vi "CCD photon image_Shaowei.vi"() -> ()   [LabVIEW 2009]
uses:
  <vilib>/Utility/file.llb/Read From Spreadsheet File (DBL).vi
  Instance           5 35Saved   CCD photon image_540_800_CR .vi
  Instance           4 35Saved   CCD photon image_540_800_CR .vi
  Instance           3 35Saved   CCD photon image_540_800_CR .vi
  Instance           8 35Saved   CCD photon image_540_800_CR .vi
  <vilib>/Analysis/Matrix/Numeric/Conversions/Array To Matrix - RA2.vi
  Instance          12 35Saved   CCD photon image_540_800_CR .vi
  Instance          18 35Saved   CCD photon image_540_800_CR .vi
  <vilib>/Analysis/Matrix/NI_Matrix.lvlib
panel:
  in  "Save Matrix6":bool
  in  "Save Matrix5":bool
  in  "Save Matrix3":bool
  in  "Save Matrix4":bool
  out "Matrix 2":string
  in  "Save Matrix2":bool
  out "Matrix 1":string
  in  "Save Matrix1":bool
  in  "select 2":bool
  in  "select":bool
  in  "next 2":bool
  in  "next":bool
  in  "previous 2":bool
  in  "previous":bool
  in  "?":bool
  out "?":path
  out "?":path
  out "?":i32
  in  "?":bool
  in  "stop 2":bool
  in  "#6":bool
  in  "#5":bool
  in  "to":dbl=950.0
  in  "From":dbl=550.0
  out "Intensity Graph 6":dbl[][](graph)
  out "Col":dbl
  out "to":dbl
  out "Matrix 6":string
  in  "lstart (nm)":dbl
  in  "lend (nm)":dbl
  out "eV":dbl
  out "eV":dbl
  out "Intensity Graph 5":dbl[][](graph)
  out "Col":dbl
  out "to":dbl
  out "Matrix 5":string
  in  "lstart (nm)":dbl
  in  "lend (nm)":dbl
  out "eV":dbl
  out "eV":dbl
  in  "?":bool
  out "MAX":dbl
  out "MIN":dbl
  out "X":sgl
  out "Y":sgl
  out "to":dbl
  out "Col":dbl
  out "eV":dbl
  out "eV":dbl
  in  "lend (nm)":dbl
  in  "lstart (nm)":dbl
  out "eV":dbl
  out "eV":dbl
  in  "lend (nm)":dbl
  in  "lstart (nm)":dbl
  out "to":dbl
  out "Col":dbl
  out "to":dbl
  out "Col":dbl
  out "eV":dbl
  out "eV":dbl
  in  "lend (nm)":dbl
  in  "lstart (nm)":dbl
  in  "?":dbl=32.0
  out "eV":dbl
  out "eV":dbl
  in  "lend (nm)":dbl
  in  "lstart (nm)":dbl
  out "to":dbl
  out "Col":dbl
  in  "#3":bool
  in  "#4":bool
  in  "#2":bool
  out "Intensity Graph 4":dbl[][](graph)
  out "Matrix 4":string
  out "Intensity Graph 3":dbl[][](graph)
  out "Matrix 3":string
  out "Intensity Graph 2":dbl[][](graph)
  out "Intensity Graph":dbl[][](graph)
  # "Input File"
  # "2 Files"
  # "1 File"
  # "1st"
  # "2nd"
  # "Spectra Range"
  # "nm"
  # "nm"
  # "# of Pixel"
  # "Image Size"
  # "Bit"
  # "Active Matrix"
  # "ON"
  # "OFF"
  # "Cosmic Ray Removal"
  # "NO"
  # "YES"
  # "Value"
  # "Position"
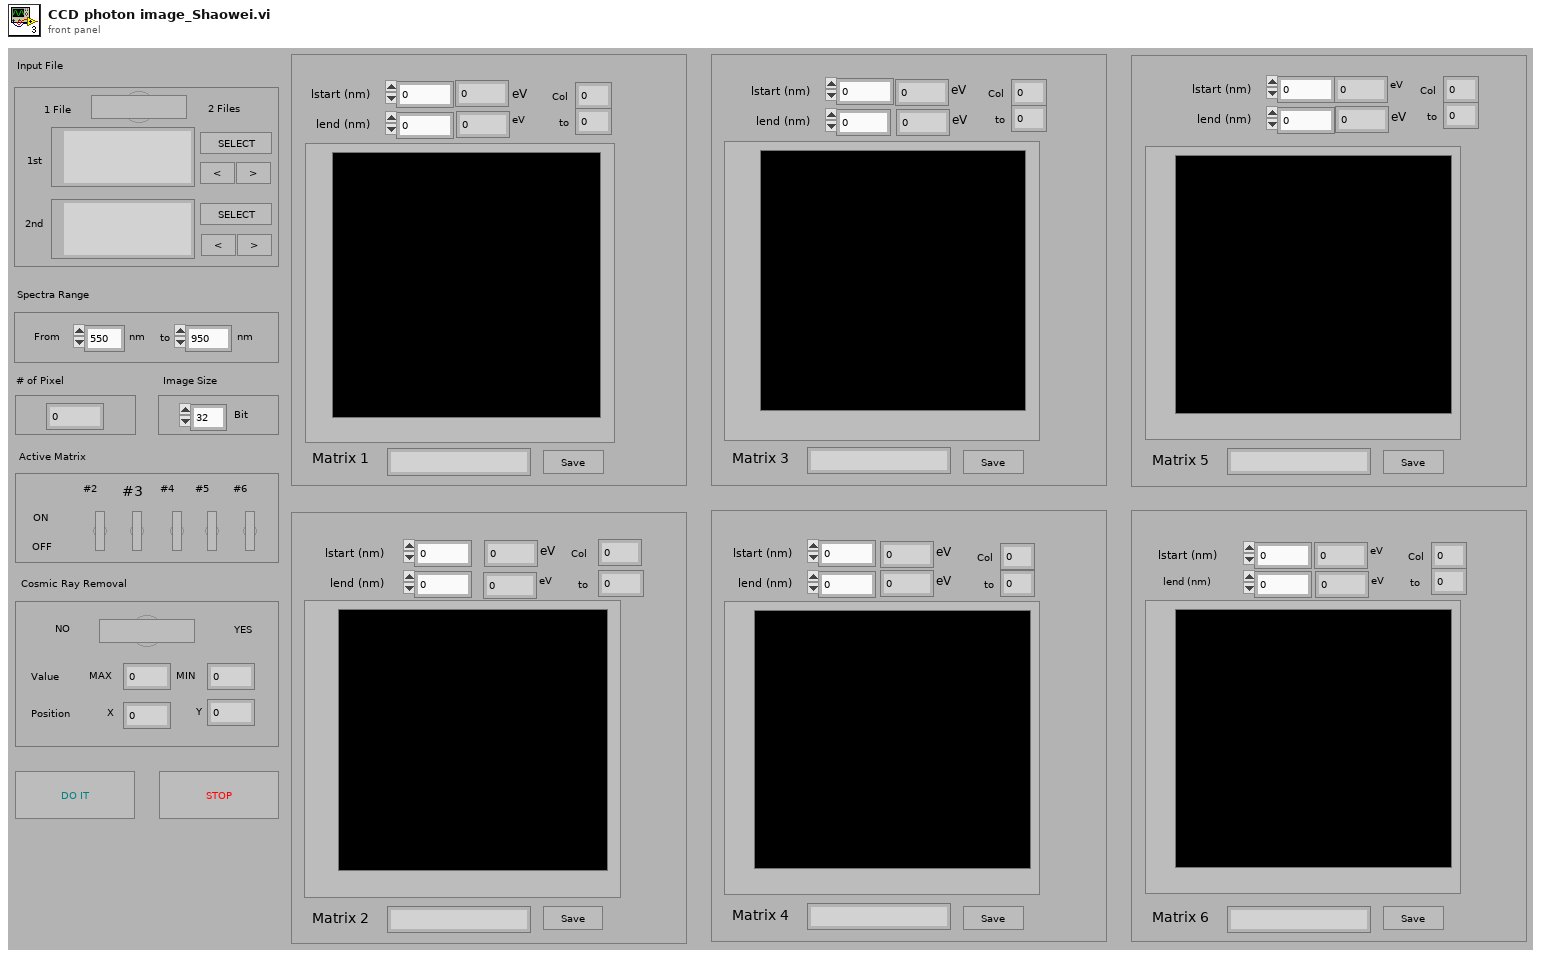
[diagram p1: front panel]
types:
  T1 = typedef "NI_Matrix.lvlib/RealMatrix.ctl" = dbl[][]
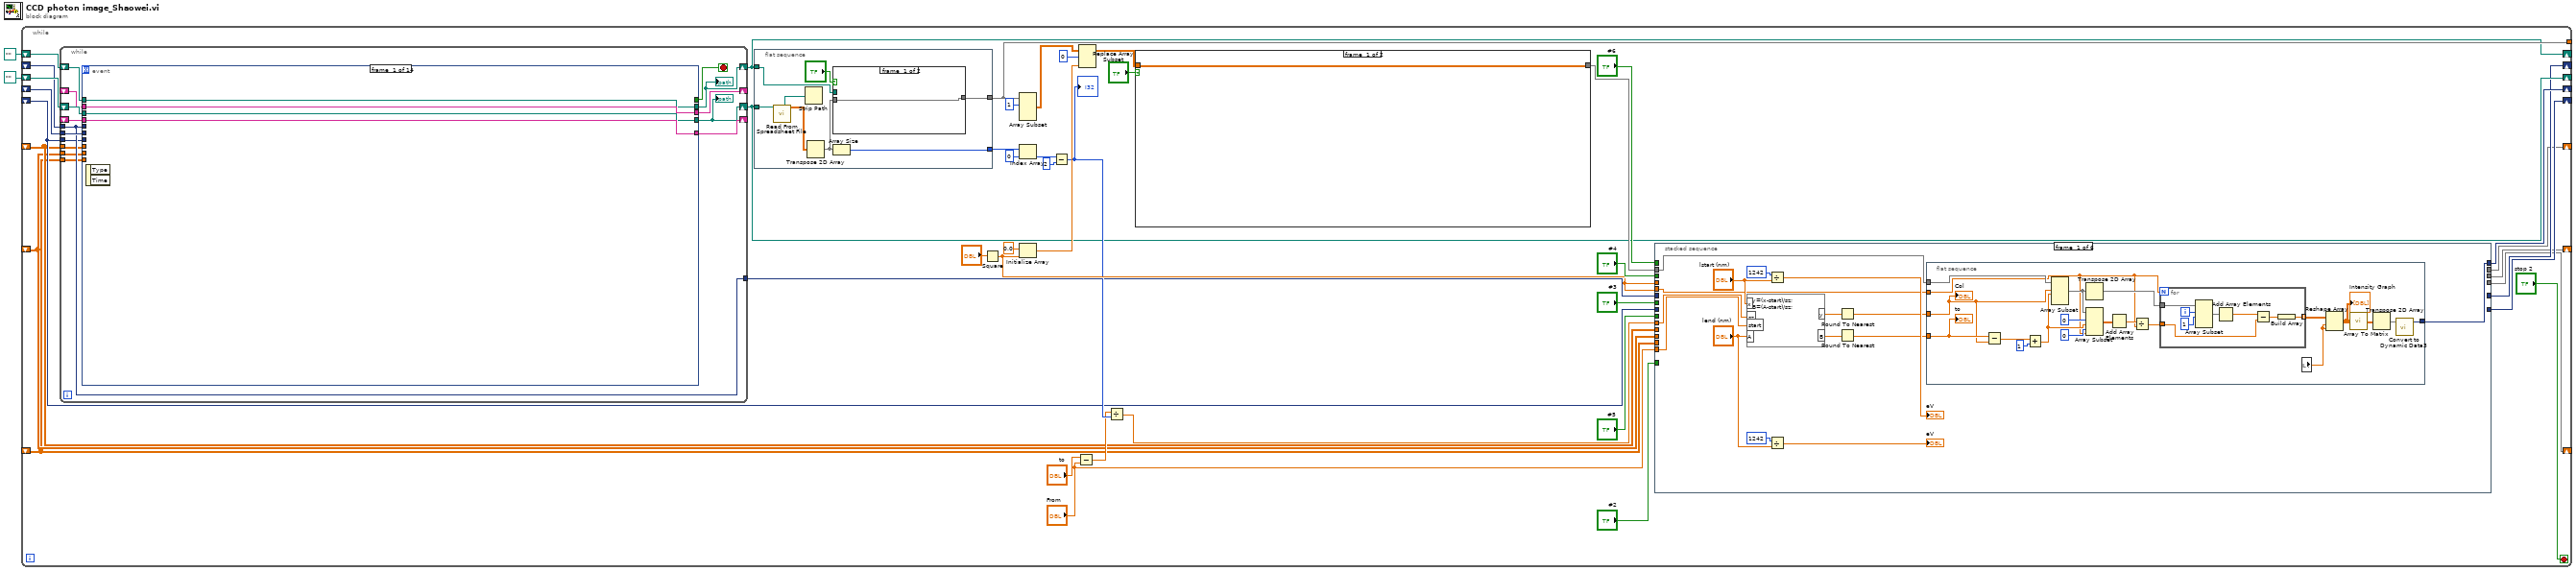
[diagram p0: block diagram]
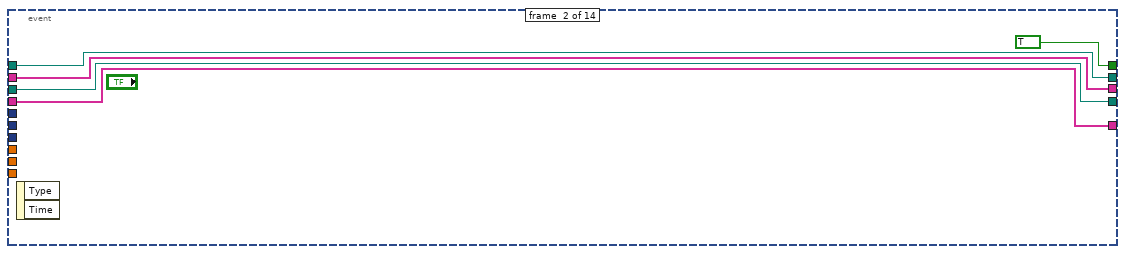
[diagram p2: hidden frame]
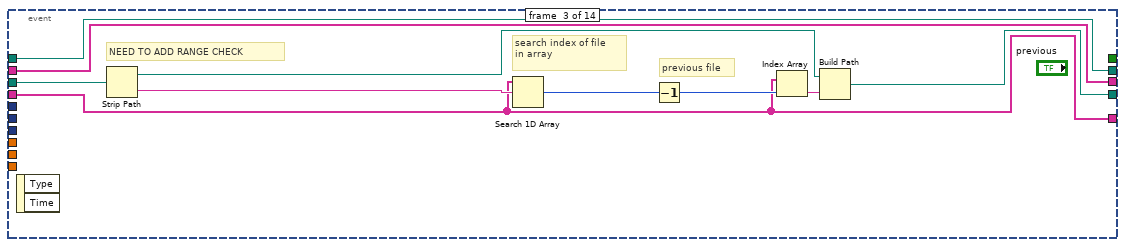
[diagram p3: hidden frame]
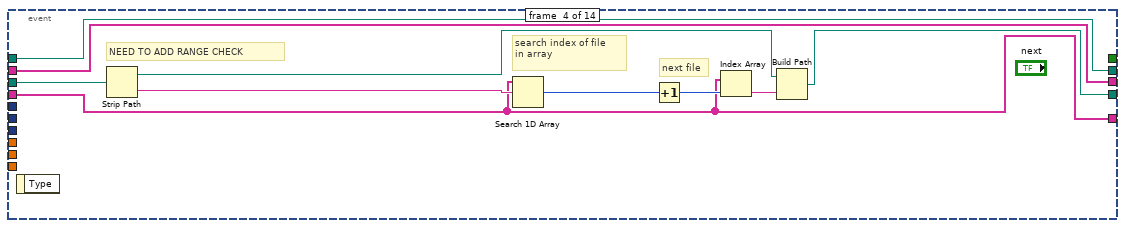
[diagram p4: hidden frame]
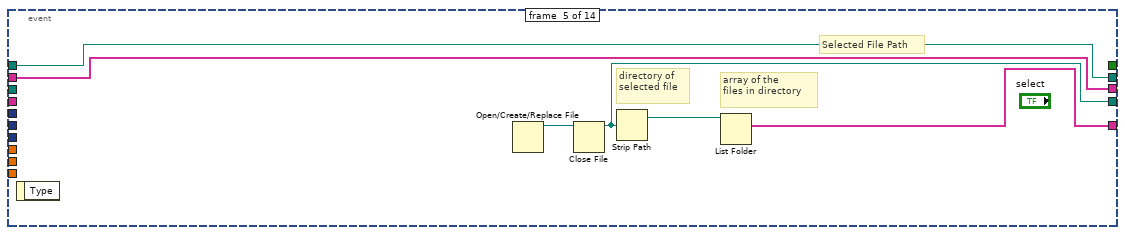
[diagram p5: hidden frame]
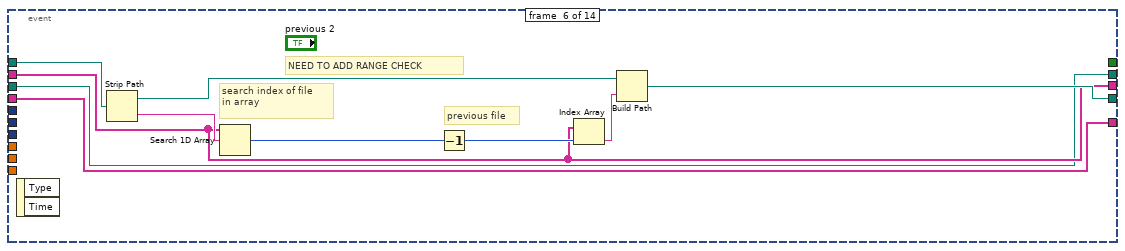
[diagram p6: hidden frame]
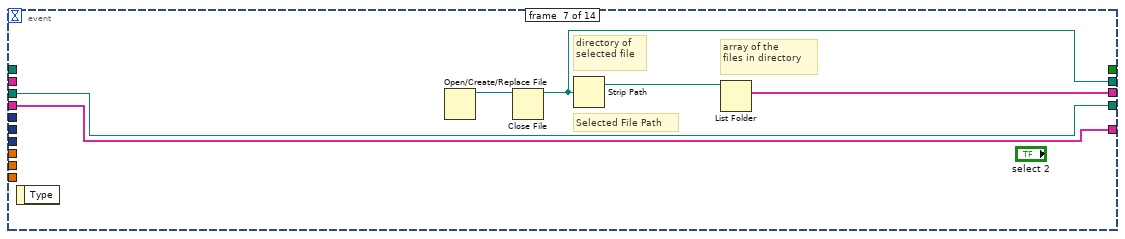
[diagram p7: hidden frame]
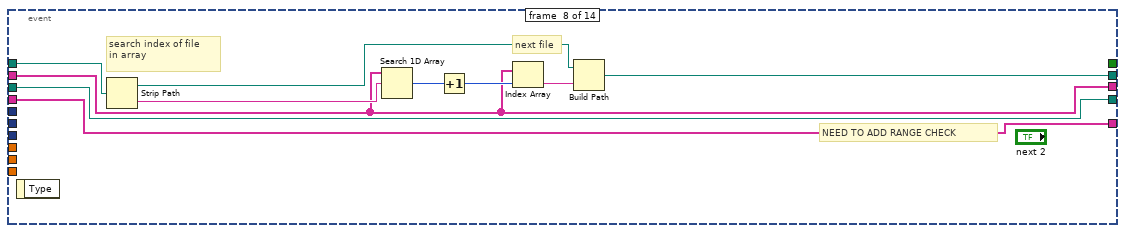
[diagram p8: hidden frame]
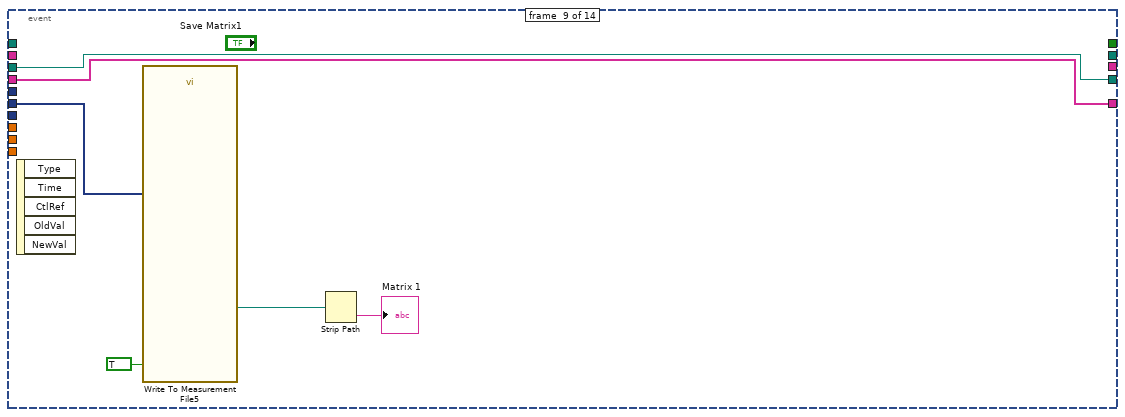
[diagram p9: hidden frame]
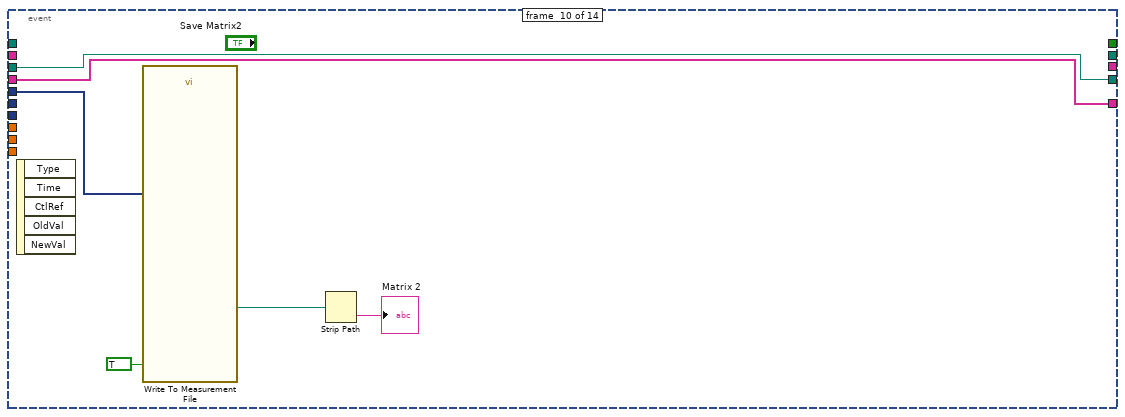
[diagram p10: hidden frame]
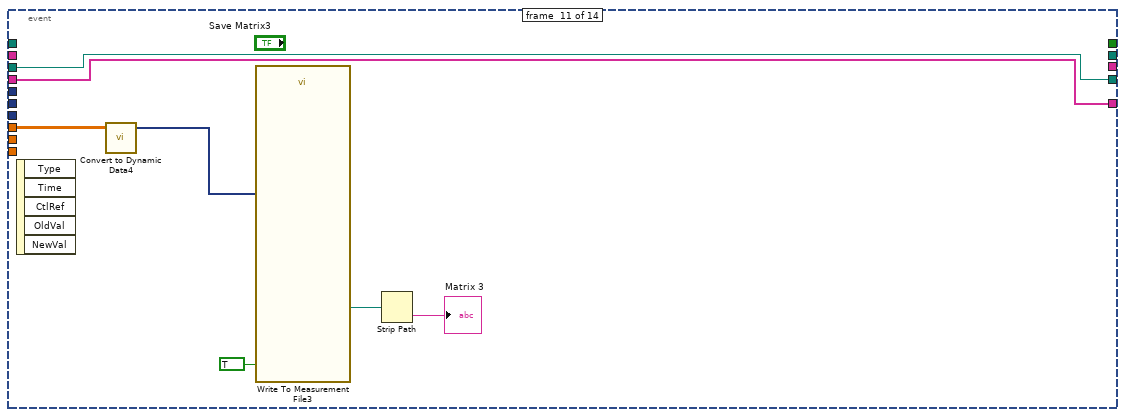
[diagram p11: hidden frame]
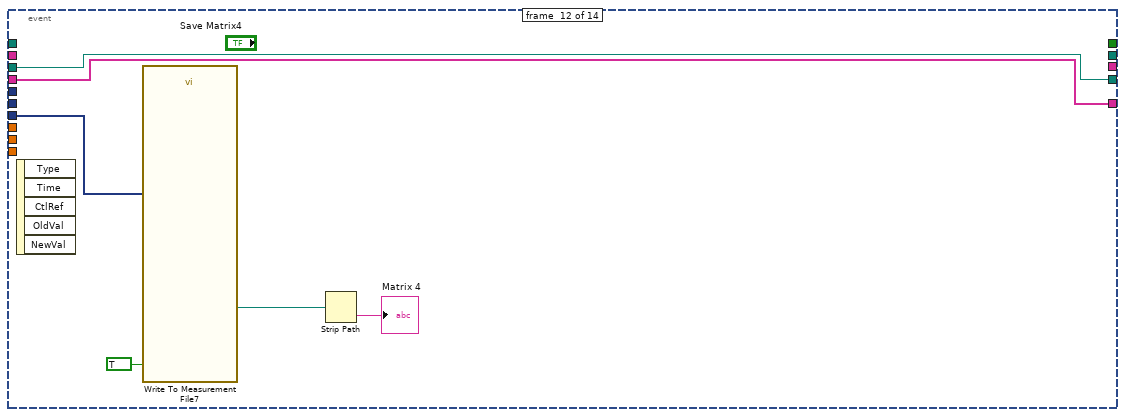
[diagram p12: hidden frame]
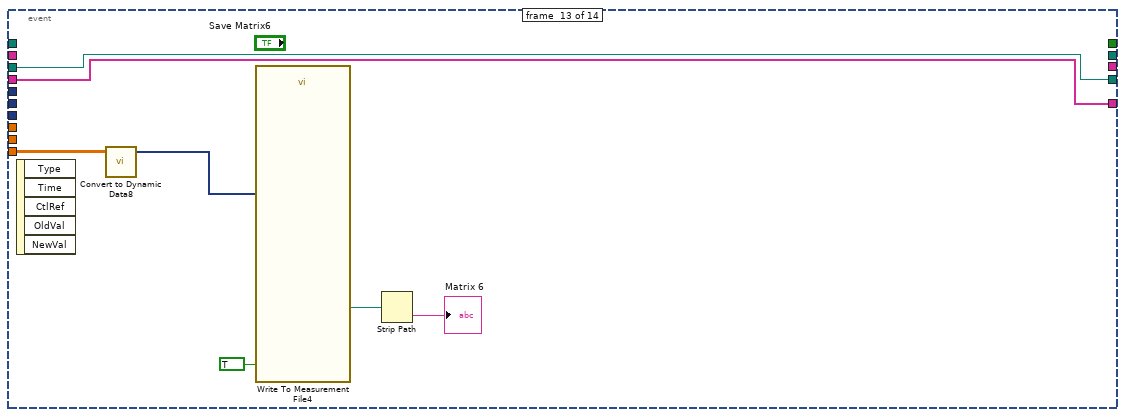
[diagram p13: hidden frame]
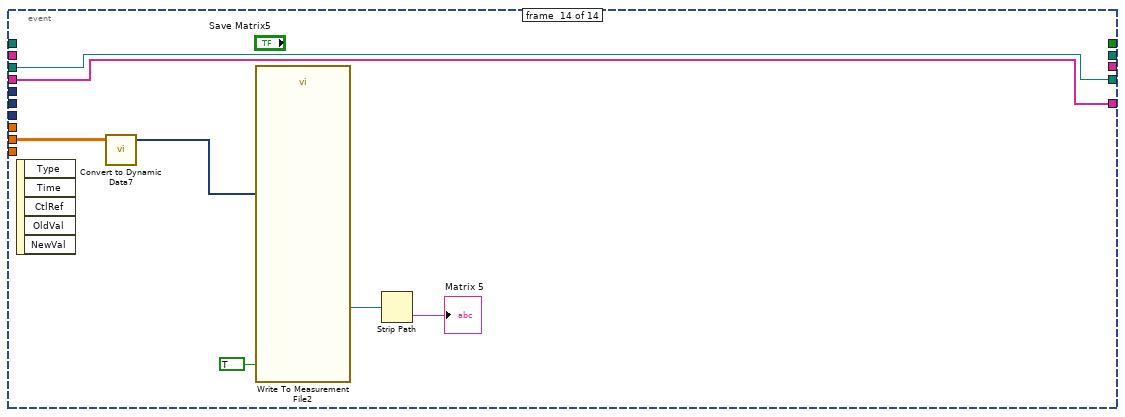
[diagram p14: hidden frame]
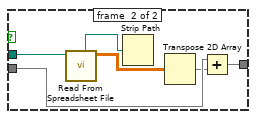
[diagram p15: hidden frame]
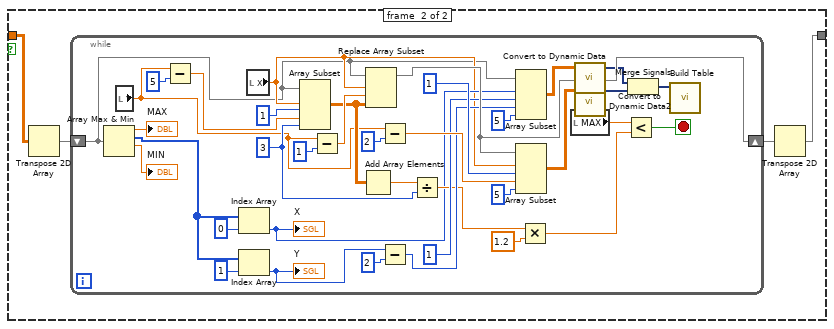
[diagram p16: hidden frame]
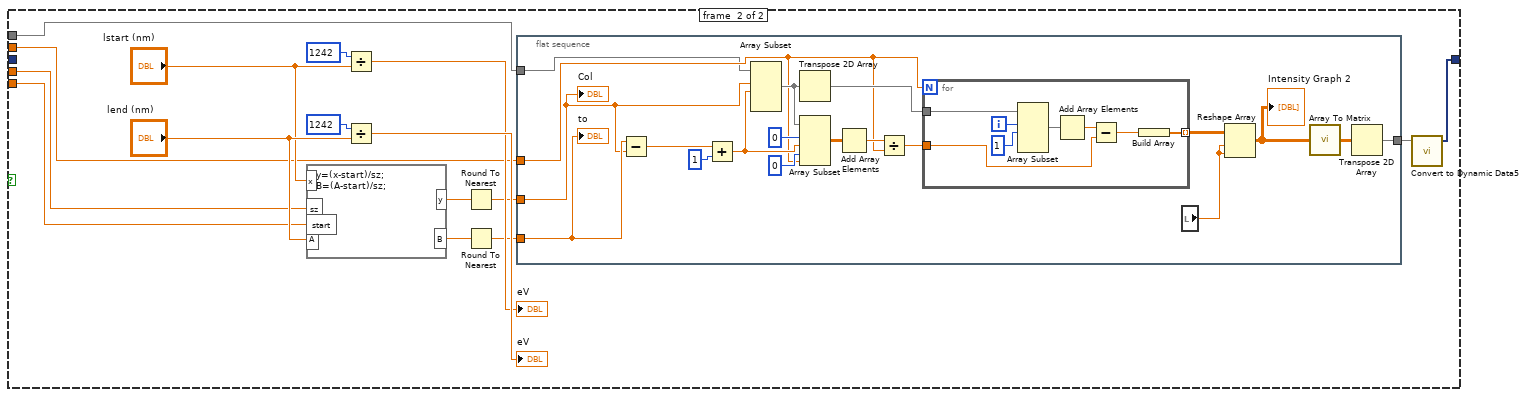
[diagram p18: hidden frame]
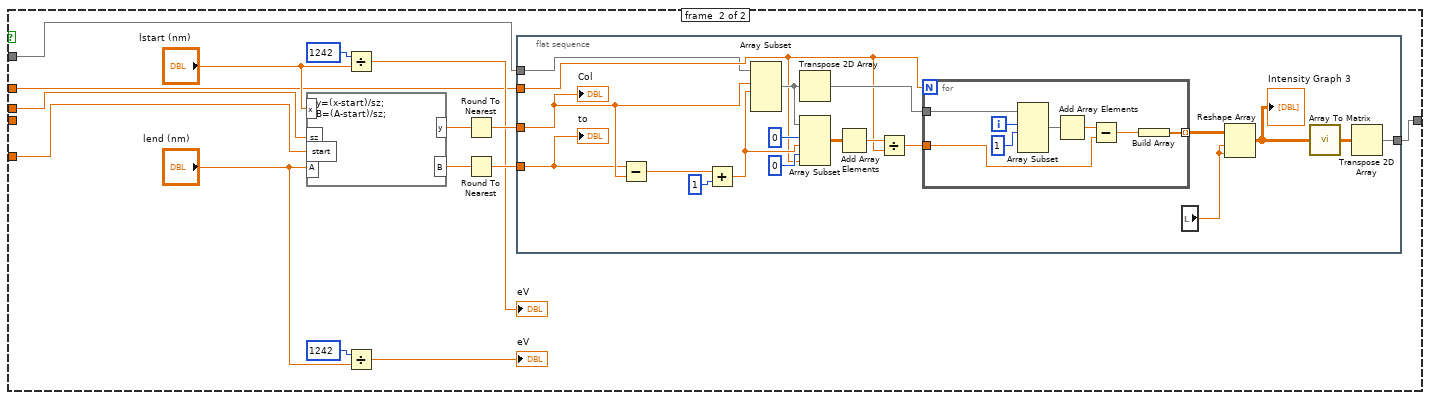
[diagram p20: hidden frame]
diagram:
  n1 = while {
    tunnel: [w26] -> _
    shift-right: [w16] -> _
    shift-left: path "" ("path") -> [w18]
    shift-right: [w17] -> _
    shift-left: path "" ("path") -> [w19]
    shift-right: [w15] -> _
    shift-left: _ -> [w14]
    shift-right: [w13] -> _
    shift-left: _ -> [w12]
    shift-right: [w10] -> _
    shift-left: _ -> [w9]
    shift-right: [w8] -> _
    shift-left: _ -> [w7]
    shift-right: [w6] -> _
    shift-left: _ -> [w5]
    shift-right: [w4] -> _
    shift-left: _ -> [w3]
    stop <- "stop 2" stop-if-true
    n2 = while {
      shift-right: [w60] -> _
      shift-left: _ -> [w59]
      shift-right: [w52] -> w16
      shift-left: w18 -> [w58]
      shift-right: [w57] -> w17
      shift-left: w19 -> [w56]
      shift-right: [w55] -> _
      shift-left: _ -> [w54]
      tunnel: w14 -> [w51]
      tunnel: w12 -> [w50]
      tunnel: [w50] -> w11
      tunnel: w9 -> [w49]
      tunnel: w7 -> [w48]
      tunnel: w5 -> [w47]
      tunnel: w3 -> [w46]
      stop <- w53 stop-if-true
      n3 = event shown="[12] \"Save Matrix6\": Value Change" {
        selector: _ -> [_ _ _ _ _ _ _ _ _ _ _ _ _ _]
        dyn-events: _ -> [_ _ _ _ _ _ _ _ _ _ _ _ _ _]
        timeout: _ -> [_ _ _ _ _ _ _ _ _ _ _ _ _ _]
        tunnel: [_ TRUE _ _ _ _ _ _ _ _ _ _ _ _] -> w53
        tunnel: [w63 w67 w72 w84 w92 w100 w107 w113 w127 w133 w140 w146 w153 w160] -> w52
        tunnel: [w64 w68 w74 w82 w93 w97 w106 w112 w126 w132 w139 w145 w152 w159] -> w60
        tunnel: w59 -> [w64 w68 w74 w82 _ w97 w106 w112 w126 w132 w139 w145 w152 w159]
        tunnel: w58 -> [w63 w67 w79 w83 _ w96 w107 w113 w127 w133 w140 w146 w153 w160]
        tunnel: [w61 w65 w70 w80 w90 w96 w109 w114 _ _ _ _ _ _] -> w57
        tunnel: w56 -> [w61 w65 w70 w80 w90 w99 _ w115 _ _ _ _ _ _]
        tunnel: [w62 w66 w71 w81 w91 w98 w108 w116 _ _ _ _ _ _] -> w55
        tunnel: w54 -> [w62 w66 w71 w81 w91 w98 _ w116 _ _ _ _ _ _]
        tunnel: w51 -> [_ _ _ _ _ _ _ _ w125 _ _ _ _ _]
        tunnel: w50 -> [_ _ _ _ _ _ _ _ _ w131 _ _ _ _]
        tunnel: w49 -> [_ _ _ _ _ _ _ _ _ _ _ w141 _ _]
        tunnel: w48 -> [_ _ _ _ _ _ _ _ _ _ w135 _ _ _]
        tunnel: w47 -> [_ _ _ _ _ _ _ _ _ _ _ _ _ w156]
        tunnel: w46 -> [_ _ _ _ _ _ _ _ _ _ _ _ w148 _]
        event #0 {
          n4 = event-data() -> ()  [unwired: 1 in, 2 out]
        }
        event #1 {
          n5 = event-data() -> ()  [unwired: 1 in, 2 out]
        }
        event #2 {
          # "NEED TO ADD RANGE CHECK"
          # "previous file"
          # "search index of file\nin array"
          n6 = event-data() -> ()  [unwired: 1 in, 2 out]
          n7 = Strip Path(path=w79) -> (stripped path=w76:path, name=w78:string)
          n8 = Search 1D Array(1D array=w74, element=w78) -> (index of element=w77:i32)  [unwired: 1 in]
          n9 = Decrement(x=w77) -> (x-1=w75:i32)
          n10 = Index Array(array=w74, index=w75) -> (element=w73:string)
          n11 = Build Path(base path=w76, name or relative path=w73) -> (appended path=w72:path)
        }
        event #3 {
          # "NEED TO ADD RANGE CHECK"
          # "next file"
          # "search index of file\nin array"
          n12 = event-data() -> ()  [unwired: 1 in, 1 out]
          n13 = Strip Path(path=w83) -> (stripped path=w87:path, name=w89:string)
          n14 = Search 1D Array(1D array=w82, element=w89) -> (index of element=w88:i32)  [unwired: 1 in]
          n15 = Increment(x=w88) -> (x+1=w86:i32)
          n16 = Index Array(array=w82, index=w86) -> (element=w85:string)
          n17 = Build Path(base path=w87, name or relative path=w85) -> (appended path=w84:path)
        }
        event #4 {
          # "array of the \nfiles in directory"
          # "directory of\nselected file"
          # "Selected File Path"
          n18 = event-data() -> ()  [unwired: 1 in, 1 out]
          n19 = Open/Create/Replace File() -> (refnum out=w95:refnum<file>)  [unwired: 6 in, 2 out]
          n20 = Close File(refnum=w95) -> (path=w92:path)  [unwired: 1 in, 1 out]
          n21 = Strip Path(path=w92) -> (stripped path=w94:path)  [unwired: 1 out]
          n22 = List Folder(path=w94) -> (filenames=w93:string[])  [unwired: 3 in, 3 out]
        }
        event #5 {
          # "NEED TO ADD RANGE CHECK"
          # "previous file"
          # "search index of file\nin array"
          n23 = event-data() -> ()  [unwired: 1 in, 2 out]
          n24 = Strip Path(path=w99) -> (stripped path=w103:path, name=w105:string)
          n25 = Search 1D Array(1D array=w98, element=w105) -> (index of element=w104:i32)  [unwired: 1 in]
          n26 = Decrement(x=w104) -> (x-1=w102:i32)
          n27 = Index Array(array=w98, index=w102) -> (element=w101:string)
          n28 = Build Path(base path=w103, name or relative path=w101) -> (appended path=w100:path)
        }
        event #6 {
          # "array of the \nfiles in directory"
          # "directory of\nselected file"
          # "Selected File Path"
          n29 = event-data() -> ()  [unwired: 1 in, 1 out]
          n30 = Open/Create/Replace File() -> (refnum out=w111:refnum<file>)  [unwired: 6 in, 2 out]
          n31 = Close File(refnum=w111) -> (path=w109:path)  [unwired: 1 in, 1 out]
          n32 = Strip Path(path=w109) -> (stripped path=w110:path)  [unwired: 1 out]
          n33 = List Folder(path=w110) -> (filenames=w108:string[])  [unwired: 3 in, 3 out]
        }
        event #7 {
          # "NEED TO ADD RANGE CHECK"
          # "next file"
          # "search index of file\nin array"
          n34 = event-data() -> ()  [unwired: 1 in, 1 out]
          n35 = Strip Path(path=w115) -> (stripped path=w119:path, name=w121:string)
          n36 = Search 1D Array(1D array=w116, element=w121) -> (index of element=w120:i32)  [unwired: 1 in]
          n37 = Increment(x=w120) -> (x+1=w118:i32)
          n38 = Index Array(array=w116, index=w118) -> (element=w117:string)
          n39 = Build Path(base path=w119, name or relative path=w117) -> (appended path=w114:path)
        }
        event #8 {
          n40 = event-data() -> ()  [unwired: 1 in, 5 out]
          n41 = call "Write To Measurement File5"("Signals"=w125, "Reset"=TRUE) -> ("Filename Out"=w123:path)  [unwired: 15 in, 2 out]
          n42 = Strip Path(path=w123) -> (name=→"Matrix 1":string)  [unwired: 1 out]
        }
        event #9 {
          n43 = event-data() -> ()  [unwired: 1 in, 5 out]
          n44 = call "Write To Measurement File"("Signals"=w131, "Reset"=TRUE) -> ("Filename Out"=w129:path)  [unwired: 15 in, 2 out]
          n45 = Strip Path(path=w129) -> (name=→"Matrix 2":string)  [unwired: 1 out]
        }
        event #10 {
          n46 = event-data() -> ()  [unwired: 1 in, 5 out]
          n47 = call "Convert to Dynamic Data4"("2D Array"=w135) -> ("Dynamic Data Type"=w134:dynamicdata)  [unwired: 3 in]
          n48 = call "Write To Measurement File3"("Signals"=w134, "Reset"=TRUE) -> ("Filename Out"=w138:path)  [unwired: 15 in, 2 out]
          n49 = Strip Path(path=w138) -> (name=→"Matrix 3":string)  [unwired: 1 out]
        }
        event #11 {
          n50 = event-data() -> ()  [unwired: 1 in, 5 out]
          n51 = call "Write To Measurement File7"("Signals"=w141, "Reset"=TRUE) -> ("Filename Out"=w143:path)  [unwired: 15 in, 2 out]
          n52 = Strip Path(path=w143) -> (name=→"Matrix 4":string)  [unwired: 1 out]
        }
        event #12 {
          n53 = event-data() -> ()  [unwired: 1 in, 5 out]
          n54 = call "Convert to Dynamic Data8"("2D Array"=w148) -> ("Dynamic Data Type"=w147:dynamicdata)  [unwired: 3 in]
          n55 = call "Write To Measurement File4"("Signals"=w147, "Reset"=TRUE) -> ("Filename Out"=w150:path)  [unwired: 15 in, 2 out]
          n56 = Strip Path(path=w150) -> (name=→"Matrix 6":string)  [unwired: 1 out]
        }
        event #13 {
          n57 = event-data() -> ()  [unwired: 1 in, 5 out]
          n58 = call "Convert to Dynamic Data7"("2D Array"=w156) -> ("Dynamic Data Type"=w155:dynamicdata)  [unwired: 3 in]
          n59 = call "Write To Measurement File2"("Signals"=w155, "Reset"=TRUE) -> ("Filename Out"=w157:path)  [unwired: 15 in, 2 out]
          n60 = Strip Path(path=w157) -> (name=→"Matrix 5":string)  [unwired: 1 out]
        }
      }
      "?" <- w52
      "?" <- w57
    }
    n61 = flat-sequence {
      tunnel: [w167] -> w26
      tunnel: [w164] -> w23
      tunnel: w16 -> [w162]
      tunnel: w17 -> [w161]
      frame #0 {
        n62 = call-poly <vilib>:"Read From Spreadsheet File.vi"("file path (dialog if empty)"=w162) -> ("all rows"=w165:dbl[][], "new file path (Not A Path if cancelled)"=w168:path)  [unwired: 6 in, 3 out]
        n63 = Strip Path(path=w168) -> ()  [unwired: 2 out]
        n64 = Transpose 2D Array(2D array=w165) -> (transposed array=w163:dbl[][])
        n65 = case shown="False" "?" {
          tunnel: w163 -> [w169 w174]
          tunnel: [w169 w173] -> w167
          tunnel: w161 -> [_ w170]
          frame #0 {
          }
          frame #1 {
            n66 = call-poly <vilib>:"Read From Spreadsheet File.vi"("file path (dialog if empty)"=w170) -> ("all rows"=w172:dbl[][], "new file path (Not A Path if cancelled)"=w175:path)  [unwired: 6 in, 3 out]
            n67 = Strip Path(path=w175) -> ()  [unwired: 2 out]
            n68 = Transpose 2D Array(2D array=w172) -> (transposed array=w171:dbl[][])
            n69 = Add(x=w174, y=w171) -> (x+y=w173:dbl[][])
          }
        }
        n70 = Array Size(array=w163) -> (size(s)=w164:i32[])
      }
    }
    n71 = Square(x="?") -> (x^2=w37:dbl)
    n72 = Array Subset(array=w26, index (row)=1) -> (w39:dbl[][])  [unwired: 3 in]
    n73 = Index Array(array=w23, index=0) -> (element=w21:i32)
    n74 = Initialize Array(0.0 ("element"), w37) -> (w41:dbl[])
    n75 = Subtract(x=w21, y=2) -> (x-y=w33:i32)
    "?" <- w33
    n76 = Subtract(x="to", y="From") -> (x-y=w32:dbl)
    n77 = Replace Array Subset(array=w39, new element=w41, index (row)=0) -> (w36:dbl[][])  [unwired: 1 in]
    n78 = Divide(x=w32, y=w33) -> (x/y=w31:dbl)
    n79 = case shown="True" "?" {
      tunnel: w36 -> [w176 w180]
      tunnel: [w176 w178] -> w35
      frame #0 {
      }
      frame #1 {
        n80 = Transpose 2D Array(2D array=w180) -> (transposed array=w179:dbl[][])
        n81 = while {
          shift-right: [w217] -> w177
          shift-left: w179 -> [w181]
          stop <- w196 stop-if-true
          w194 = 3
          n82 = Array Max & Min(array=w181) -> (max value=→"MAX":dbl, max index (indices)=w215:i32[], min value=→"MIN":dbl)  [unwired: 1 out]
          n83 = local read "Y"() -> (w183:sgl)
          n84 = Subtract(x=w183, y=5) -> (x-y=w211:sgl)
          n85 = Index Array(array=w215, index=0) -> (element=w188:i32)
          "X" <- w188
          n86 = Index Array(array=w215, index=1) -> (element=w187:i32)
          "Y" <- w187
          n87 = local read "X"() -> (w184:sgl)
          n88 = Array Subset(array=w181, index (row)=w184, length (row)=1, index (col)=w211, length (col)=w194) -> (w193:dbl[][])
          n89 = Subtract(x=w183, y=1) -> (x-y=w210:sgl)
          n90 = Add Array Elements(numeric array=w193) -> (sum=w195:dbl)
          n91 = Replace Array Subset(array=w181, new element=w193, index (row)=w184, index (col)=w210) -> (w217:dbl[][])
          n92 = Subtract(x=w183, y=2) -> (x-y=w206:sgl)
          n93 = Subtract(x=w187, y=2) -> (x-y=w201:i32)
          n94 = Divide(x=w195, y=w194) -> (x/y=w192:dbl)
          n95 = Array Subset(array=w181, index (row)=w188, length (row)=1, index (col)=w201, length (col)=5) -> (w199:dbl[][])
          n96 = Array Subset(array=w217, index (row)=w184, length (row)=1, index (col)=w206, length (col)=5) -> (w204:dbl[][])
          n97 = Multiply(x=w192, y=1.2) -> (x*y=w197:dbl)
          n98 = local read "MAX"() -> (w182:dbl)
          n99 = call "Convert to Dynamic Data"("2D Array"=w199) -> ("Dynamic Data Type"=w191:dynamicdata)  [unwired: 3 in]
          n100 = call "Convert to Dynamic Data2"("2D Array"=w204) -> ("Dynamic Data Type"=w189:dynamicdata)  [unwired: 3 in]
          n101 = Less?(x=w182, y=w197) -> (x < y?=w196:bool)
          n102 = Merge Signals(w191, w189) -> (w190:dynamicdata)
          n103 = call "Build Table"("Signals"=w190) -> ()  [unwired: 9 in, 2 out]
        }
        n104 = Transpose 2D Array(2D array=w177) -> (transposed array=w178:dbl[][])
      }
    }
    n105 = stacked-sequence {
      tunnel: "#4" -> [_ _ _ w368 _ _]
      tunnel: "#3" -> [_ _ w318 _ _ _]
      tunnel: "#2" -> [_ w267 _ _ _ _]
      tunnel: w37 -> [w222 w266 w317 _ _ _]
      tunnel: w35 -> [w221 w265 w316 w366 w418 w468]
      tunnel: w37 -> [_ _ _ w367 w419 w469]
      tunnel: w31 -> [w220 w264 w315 w364 w417 w467]
      tunnel: "From" -> [w219 w263 w314 w365 w416 w466]
      tunnel: "#5" -> [_ _ _ _ w415 _]
      tunnel: "#6" -> [_ _ _ _ _ w465]
      tunnel: [w218 _ _ _ _ _] -> w15
      tunnel: [_ w262 _ _ _ _] -> w13
      tunnel: w11 -> [_ w261 _ _ _ _]
      tunnel: [_ _ _ w363 _ _] -> w10
      tunnel: w9 -> [_ _ _ w362 _ _]
      tunnel: [_ _ w313 _ _ _] -> w8
      tunnel: w7 -> [_ _ w312 _ _ _]
      tunnel: [_ _ _ _ w414 _] -> w6
      tunnel: w5 -> [_ _ _ _ w413 _]
      tunnel: [_ _ _ _ _ w464] -> w4
      tunnel: w3 -> [_ _ _ _ _ w463]
      frame #0 {
        n106 = formula code="y=(x-start)/sz;\nB=(A-start)/sz;"("x"="lstart (nm)", "A"="lend (nm)", "sz"=w220, "start"=w219) -> ("y"=w226:dbl, "B"=w225:dbl)
        n107 = Divide(x=1242, y="lstart (nm)") -> (x/y=→"eV":dbl)
        n108 = Divide(x=1242, y="lend (nm)") -> (x/y=→"eV":dbl)
        n109 = Round To Nearest(number=w226) -> (nearest integer value=w224:dbl)
        n110 = Round To Nearest(number=w225) -> (nearest integer value=w223:dbl)
        n111 = flat-sequence {
          tunnel: [w252] -> w218
          tunnel: w223 -> [w245]
          tunnel: w224 -> [w244]
          tunnel: w222 -> [w233]
          tunnel: w221 -> [w237]
          frame #0 {
            n112 = Subtract(x=w245, y=w244) -> (x-y=w240:dbl)
            n113 = Add(x=w240, y=1) -> (x+y=w238:dbl)
            n114 = Array Subset(array=w237, index (row)=w244, length (row)=w238) -> (w236:dbl[][])  [unwired: 2 in]
            n115 = Transpose 2D Array(2D array=w236) -> (transposed array=w247:dbl[][])
            n116 = Array Subset(array=w236, index (row)=0, length (row)=w238, index (col)=0, length (col)=w233) -> (w235:dbl[][])
            n117 = Add Array Elements(numeric array=w235) -> (sum=w241:dbl)
            n118 = Divide(x=w241, y=w233) -> (x/y=w239:dbl)
            n119 = for {
              N: w233 -> [_]
              tunnel: w247 -> [w254]
              tunnel: [w256] -> w246 mode=indexing
              tunnel: w239 -> [w255]
              i -> [w260]
              n120 = Array Subset(array=w254, index (row)=w260, length (row)=1) -> (w253:dbl[][])  [unwired: 2 in]
              n121 = Add Array Elements(numeric array=w253) -> (sum=w258:dbl)
              n122 = Subtract(x=w258, y=w255) -> (x-y=w257:dbl)
              n123 = Build Array(w257) -> (w256:dbl[])
            }
            n124 = local read item#15() -> (w234:dbl)
            n125 = Reshape Array(w246, w234, w234) -> (w248:dbl[][])
            "Intensity Graph" <- w248
            n126 = call-poly <vilib>:"Array To Matrix.vi"("Real 2D Array"=w248) -> ("Real Matrix"=w251:T1)
            n127 = Transpose 2D Array(2D array=w251) -> (transposed array=w250:T1)
            n128 = call "Convert to Dynamic Data3"("2D Array"=w250) -> ("Dynamic Data Type"=w252:dynamicdata)  [unwired: 3 in]
            "Col" <- w244
            "to" <- w245
          }
        }
      }
      frame #1 {
        n129 = case shown="True" w267 {
          tunnel: w266 -> [_ w274]
          tunnel: w265 -> [_ w273]
          tunnel: w264 -> [_ w272]
          tunnel: w263 -> [_ w271]
          tunnel: [w268 w269] -> w262
          tunnel: w261 -> [w268 _]
          frame #0 {
          }
          frame #1 {
            n130 = formula code="y=(x-start)/sz;\nB=(A-start)/sz;"("x"="lstart (nm)", "A"="lend (nm)", "sz"=w272, "start"=w271) -> ("y"=w278:dbl, "B"=w277:dbl)
            n131 = Divide(x=1242, y="lstart (nm)") -> (x/y=→"eV":dbl)
            n132 = Divide(x=1242, y="lend (nm)") -> (x/y=→"eV":dbl)
            n133 = Round To Nearest(number=w278) -> (nearest integer value=w276:dbl)
            n134 = Round To Nearest(number=w277) -> (nearest integer value=w275:dbl)
            n135 = flat-sequence {
              tunnel: w276 -> [w290]
              tunnel: w275 -> [w291]
              tunnel: [w298] -> w270
              tunnel: w274 -> [w286]
              tunnel: w273 -> [w285]
              frame #0 {
                n136 = Subtract(x=w291, y=w290) -> (x-y=w299:dbl)
                n137 = Add(x=w299, y=1) -> (x+y=w293:dbl)
                n138 = Array Subset(array=w285, index (row)=w290, length (row)=w293) -> (w289:dbl[][])  [unwired: 2 in]
                n139 = Transpose 2D Array(2D array=w289) -> (transposed array=w302:dbl[][])
                n140 = Array Subset(array=w289, index (row)=0, length (row)=w293, index (col)=0, length (col)=w286) -> (w287:dbl[][])
                n141 = Add Array Elements(numeric array=w287) -> (sum=w296:dbl)
                n142 = Divide(x=w296, y=w286) -> (x/y=w292:dbl)
                n143 = for {
                  N: w286 -> [_]
                  tunnel: w302 -> [w311]
                  tunnel: [w304] -> w303 mode=indexing
                  tunnel: w292 -> [w306]
                  i -> [w310]
                  n144 = Array Subset(array=w311, index (row)=w310, length (row)=1) -> (w309:dbl[][])  [unwired: 2 in]
                  n145 = Add Array Elements(numeric array=w309) -> (sum=w307:dbl)
                  n146 = Subtract(x=w307, y=w306) -> (x-y=w305:dbl)
                  n147 = Build Array(w305) -> (w304:dbl[])
                }
                n148 = local read item#15() -> (w288:dbl)
                n149 = Reshape Array(w303, w288, w288) -> (w301:dbl[][])
                "Intensity Graph 2" <- w301
                n150 = call-poly <vilib>:"Array To Matrix.vi"("Real 2D Array"=w301) -> ("Real Matrix"=w297:T1)
                n151 = Transpose 2D Array(2D array=w297) -> (transposed array=w298:T1)
                "Col" <- w290
                "to" <- w291
              }
            }
            n152 = call "Convert to Dynamic Data5"("2D Array"=w270) -> ("Dynamic Data Type"=w269:dynamicdata)  [unwired: 3 in]
          }
        }
      }
      frame #2 {
        n153 = case shown="False" w318 {
          tunnel: w317 -> [_ w324]
          tunnel: w316 -> [_ w323]
          tunnel: w315 -> [_ w322]
          tunnel: w314 -> [_ w321]
          tunnel: [w319 w320] -> w313
          tunnel: w312 -> [w319 _]
          frame #0 {
          }
          frame #1 {
            n154 = formula code="y=(x-start)/sz;\nB=(A-start)/sz;"("x"="lstart (nm)", "A"="lend (nm)", "sz"=w322, "start"=w321) -> ("y"=w332:dbl, "B"=w331:dbl)
            n155 = Divide(x=1242, y="lstart (nm)") -> (x/y=→"eV":dbl)
            n156 = Divide(x=1242, y="lend (nm)") -> (x/y=→"eV":dbl)
            n157 = Round To Nearest(number=w332) -> (nearest integer value=w330:dbl)
            n158 = Round To Nearest(number=w331) -> (nearest integer value=w329:dbl)
            n159 = flat-sequence {
              tunnel: w329 -> [w340]
              tunnel: w330 -> [w341]
              tunnel: [w348] -> w320
              tunnel: w324 -> [w336]
              tunnel: w323 -> [w335]
              frame #0 {
                n160 = Subtract(x=w340, y=w341) -> (x-y=w349:dbl)
                n161 = Add(x=w349, y=1) -> (x+y=w343:dbl)
                n162 = Array Subset(array=w335, index (row)=w341, length (row)=w343) -> (w337:dbl[][])  [unwired: 2 in]
                n163 = Transpose 2D Array(2D array=w337) -> (transposed array=w352:dbl[][])
                n164 = Array Subset(array=w337, index (row)=0, length (row)=w343, index (col)=0, length (col)=w336) -> (w338:dbl[][])
                n165 = Add Array Elements(numeric array=w338) -> (sum=w344:dbl)
                n166 = Divide(x=w344, y=w336) -> (x/y=w342:dbl)
                n167 = for {
                  N: w336 -> [_]
                  tunnel: w352 -> [w361]
                  tunnel: [w355] -> w353 mode=indexing
                  tunnel: w342 -> [w354]
                  i -> [w360]
                  n168 = Array Subset(array=w361, index (row)=w360, length (row)=1) -> (w359:dbl[][])  [unwired: 2 in]
                  n169 = Add Array Elements(numeric array=w359) -> (sum=w357:dbl)
                  n170 = Subtract(x=w357, y=w354) -> (x-y=w356:dbl)
                  n171 = Build Array(w356) -> (w355:dbl[])
                }
                n172 = local read item#15() -> (w339:dbl)
                n173 = Reshape Array(w353, w339, w339) -> (w351:dbl[][])
                "Intensity Graph 3" <- w351
                n174 = call-poly <vilib>:"Array To Matrix.vi"("Real 2D Array"=w351) -> ("Real Matrix"=w347:T1)
                n175 = Transpose 2D Array(2D array=w347) -> (transposed array=w348:T1)
                "Col" <- w341
                "to" <- w340
              }
            }
          }
        }
      }
      frame #3 {
        n176 = case shown="False" w368 {
          tunnel: w367 -> [_ w375]
          tunnel: w366 -> [_ w374]
          tunnel: w365 -> [_ w373]
          tunnel: w364 -> [_ w372]
          tunnel: [w369 w370] -> w363
          tunnel: w362 -> [w369 _]
          frame #0 {
          }
          frame #1 {
            n177 = formula code="y=(x-start)/sz;\nB=(A-start)/sz;"("x"="lstart (nm)", "A"="lend (nm)", "sz"=w372, "start"=w373) -> ("y"=w383:dbl, "B"=w382:dbl)
            n178 = Divide(x=1242, y="lstart (nm)") -> (x/y=→"eV":dbl)
            n179 = Divide(x=1242, y="lend (nm)") -> (x/y=→"eV":dbl)
            n180 = Round To Nearest(number=w383) -> (nearest integer value=w377:dbl)
            n181 = Round To Nearest(number=w382) -> (nearest integer value=w376:dbl)
            n182 = flat-sequence {
              tunnel: w377 -> [w393]
              tunnel: w376 -> [w392]
              tunnel: [w400] -> w371
              tunnel: w375 -> [w386]
              tunnel: w374 -> [w387]
              frame #0 {
                n183 = Subtract(x=w392, y=w393) -> (x-y=w401:dbl)
                n184 = Add(x=w401, y=1) -> (x+y=w394:dbl)
                n185 = Array Subset(array=w387, index (row)=w393, length (row)=w394) -> (w391:dbl[][])  [unwired: 2 in]
                n186 = Transpose 2D Array(2D array=w391) -> (transposed array=w390:dbl[][])
                n187 = Array Subset(array=w391, index (row)=0, length (row)=w394, index (col)=0, length (col)=w386) -> (w388:dbl[][])
                n188 = Add Array Elements(numeric array=w388) -> (sum=w396:dbl)
                n189 = Divide(x=w396, y=w386) -> (x/y=w395:dbl)
                n190 = for {
                  N: w386 -> [_]
                  tunnel: w390 -> [w412]
                  tunnel: [w406] -> w404 mode=indexing
                  tunnel: w395 -> [w405]
                  i -> [w411]
                  n191 = Array Subset(array=w412, index (row)=w411, length (row)=1) -> (w410:dbl[][])  [unwired: 2 in]
                  n192 = Add Array Elements(numeric array=w410) -> (sum=w408:dbl)
                  n193 = Subtract(x=w408, y=w405) -> (x-y=w407:dbl)
                  n194 = Build Array(w407) -> (w406:dbl[])
                }
                n195 = local read item#15() -> (w389:dbl)
                n196 = Reshape Array(w404, w389, w389) -> (w403:dbl[][])
                "Intensity Graph 4" <- w403
                n197 = call-poly <vilib>:"Array To Matrix.vi"("Real 2D Array"=w403) -> ("Real Matrix"=w399:T1)
                n198 = Transpose 2D Array(2D array=w399) -> (transposed array=w400:T1)
                "Col" <- w393
                "to" <- w392
              }
            }
            n199 = call "Convert to Dynamic Data6"("2D Array"=w371) -> ("Dynamic Data Type"=w370:dynamicdata)  [unwired: 3 in]
          }
        }
      }
      frame #4 {
        n200 = case shown="False" w415 {
          tunnel: w419 -> [_ w425]
          tunnel: w418 -> [_ w424]
          tunnel: w417 -> [_ w423]
          tunnel: w416 -> [_ w422]
          tunnel: [w420 w421] -> w414
          tunnel: w413 -> [w420 _]
          frame #0 {
          }
          frame #1 {
            n201 = formula code="y=(x-start)/sz;\nB=(A-start)/sz;"("x"="lstart (nm)", "A"="lend (nm)", "sz"=w423, "start"=w422) -> ("y"=w433:dbl, "B"=w432:dbl)
            n202 = Divide(x=1242, y="lstart (nm)") -> (x/y=→"eV":dbl)
            n203 = Divide(x=1242, y="lend (nm)") -> (x/y=→"eV":dbl)
            n204 = Round To Nearest(number=w433) -> (nearest integer value=w427:dbl)
            n205 = Round To Nearest(number=w432) -> (nearest integer value=w426:dbl)
            n206 = flat-sequence {
              tunnel: w427 -> [w443]
              tunnel: w426 -> [w442]
              tunnel: [w450] -> w421
              tunnel: w425 -> [w436]
              tunnel: w424 -> [w437]
              frame #0 {
                n207 = Subtract(x=w442, y=w443) -> (x-y=w451:dbl)
                n208 = Add(x=w451, y=1) -> (x+y=w444:dbl)
                n209 = Array Subset(array=w437, index (row)=w443, length (row)=w444) -> (w441:dbl[][])  [unwired: 2 in]
                n210 = Transpose 2D Array(2D array=w441) -> (transposed array=w440:dbl[][])
                n211 = Array Subset(array=w441, index (row)=0, length (row)=w444, index (col)=0, length (col)=w436) -> (w438:dbl[][])
                n212 = Add Array Elements(numeric array=w438) -> (sum=w446:dbl)
                n213 = Divide(x=w446, y=w436) -> (x/y=w445:dbl)
                n214 = for {
                  N: w436 -> [_]
                  tunnel: w440 -> [w462]
                  tunnel: [w456] -> w454 mode=indexing
                  tunnel: w445 -> [w455]
                  i -> [w461]
                  n215 = Array Subset(array=w462, index (row)=w461, length (row)=1) -> (w460:dbl[][])  [unwired: 2 in]
                  n216 = Add Array Elements(numeric array=w460) -> (sum=w458:dbl)
                  n217 = Subtract(x=w458, y=w455) -> (x-y=w457:dbl)
                  n218 = Build Array(w457) -> (w456:dbl[])
                }
                n219 = local read item#15() -> (w439:dbl)
                n220 = Reshape Array(w454, w439, w439) -> (w453:dbl[][])
                "Intensity Graph 5" <- w453
                n221 = call-poly <vilib>:"Array To Matrix.vi"("Real 2D Array"=w453) -> ("Real Matrix"=w449:T1)
                n222 = Transpose 2D Array(2D array=w449) -> (transposed array=w450:T1)
                "Col" <- w443
                "to" <- w442
              }
            }
          }
        }
      }
      frame #5 {
        n223 = case shown="False" w465 {
          tunnel: w469 -> [_ w475]
          tunnel: w468 -> [_ w474]
          tunnel: w467 -> [_ w473]
          tunnel: w466 -> [_ w472]
          tunnel: [w470 w471] -> w464
          tunnel: w463 -> [w470 _]
          frame #0 {
          }
          frame #1 {
            n224 = formula code="y=(x-start)/sz;\nB=(A-start)/sz;"("x"="lstart (nm)", "A"="lend (nm)", "sz"=w473, "start"=w472) -> ("y"=w483:dbl, "B"=w482:dbl)
            n225 = Divide(x=1242, y="lstart (nm)") -> (x/y=→"eV":dbl)
            n226 = Divide(x=1242, y="lend (nm)") -> (x/y=→"eV":dbl)
            n227 = Round To Nearest(number=w483) -> (nearest integer value=w477:dbl)
            n228 = Round To Nearest(number=w482) -> (nearest integer value=w476:dbl)
            n229 = flat-sequence {
              tunnel: w477 -> [w493]
              tunnel: w476 -> [w492]
              tunnel: [w500] -> w471
              tunnel: w475 -> [w486]
              tunnel: w474 -> [w487]
              frame #0 {
                n230 = Subtract(x=w492, y=w493) -> (x-y=w501:dbl)
                n231 = Add(x=w501, y=1) -> (x+y=w494:dbl)
                n232 = Array Subset(array=w487, index (row)=w493, length (row)=w494) -> (w491:dbl[][])  [unwired: 2 in]
                n233 = Transpose 2D Array(2D array=w491) -> (transposed array=w490:dbl[][])
                n234 = Array Subset(array=w491, index (row)=0, length (row)=w494, index (col)=0, length (col)=w486) -> (w488:dbl[][])
                n235 = Add Array Elements(numeric array=w488) -> (sum=w496:dbl)
                n236 = Divide(x=w496, y=w486) -> (x/y=w495:dbl)
                n237 = for {
                  N: w486 -> [_]
                  tunnel: w490 -> [w512]
                  tunnel: [w506] -> w504 mode=indexing
                  tunnel: w495 -> [w505]
                  i -> [w511]
                  n238 = Array Subset(array=w512, index (row)=w511, length (row)=1) -> (w510:dbl[][])  [unwired: 2 in]
                  n239 = Add Array Elements(numeric array=w510) -> (sum=w508:dbl)
                  n240 = Subtract(x=w508, y=w505) -> (x-y=w507:dbl)
                  n241 = Build Array(w507) -> (w506:dbl[])
                }
                n242 = local read item#15() -> (w489:dbl)
                n243 = Reshape Array(w504, w489, w489) -> (w503:dbl[][])
                "Intensity Graph 6" <- w503
                n244 = call-poly <vilib>:"Array To Matrix.vi"("Real 2D Array"=w503) -> ("Real Matrix"=w499:T1)
                n245 = Transpose 2D Array(2D array=w499) -> (transposed array=w500:T1)
                "Col" <- w493
                "to" <- w492
              }
            }
          }
        }
      }
    }
  }
